vi "Traj_constraint_encapsulate.vi"() -> ()   [LabVIEW 2019]
uses:
  <vilib>/Utility/Data Type/Type Definitions/Data Type.ctl
  <vilib>/Utility/Data Type/Type Definitions/Type Definition Info.ctl
  <vilib>/Rock Robotics/WPI/ThirdParty/JAS_Junk/TrajLib/POSE2D.ctl
  <vilib>/Rock Robotics/WPI/ThirdParty/JAS_Junk/TrajLib/TRANSLATION2D.ctl
  <vilib>/Rock Robotics/WPI/ThirdParty/JAS_Junk/TrajLib/ROTATION2D.ctl
  <vilib>/Rock Robotics/WPI/ThirdParty/JAS_Junk/TrajLib/SIMPLE_MOTOR_FF.ctl
  <vilib>/Rock Robotics/WPI/ThirdParty/JAS_Junk/TrajLib/TRAJ_CONSTRAINT_DIIF_DRIVE_KINEMATICS.ctl
  <vilib>/Rock Robotics/WPI/ThirdParty/JAS_Junk/TrajLib/DIFF_DRIVE_KINEMATICS.ctl
  <vilib>/Rock Robotics/WPI/ThirdParty/JAS_Junk/TrajLib/TRAJ_CONSTRAINT_CENTRIPETAL_ACCEL.ctl
  <vilib>/Rock Robotics/WPI/ThirdParty/JAS_Junk/TrajLib/TRAJ_CONSTRAINT_DIIF_DRIVE_VOLTAGE.ctl
  <vilib>/Rock Robotics/WPI/ThirdParty/JAS_Junk/TrajLib/TRAJ_CONSTRAINT_MECA_DRIVE_KINEMATICS.ctl
  <vilib>/Rock Robotics/WPI/ThirdParty/JAS_Junk/TrajLib/MECA_DRIVE_KINEMATICS.ctl
  <vilib>/Analysis/Matrix/Datatypes/RealMatrix.ctl
  <vilib>/Rock Robotics/WPI/ThirdParty/JAS_Junk/TrajLib/TRAJ_CONSTRAINT_SWERVE_DRIVE_KINEMATICS.ctl
  <vilib>/Rock Robotics/WPI/ThirdParty/JAS_Junk/TrajLib/SWERVE_DRIVE_KINEMATICS.ctl
  <vilib>/Rock Robotics/SystemInterfaces/NetworkCommunication/NetComm_UsageReport_report.vi
  <vilib>/Rock Robotics/WPI/ThirdParty/JAS_Junk/TrajLib/Util_LibraryGlobals.vi
  <vilib>/Rock Robotics/WPI/ThirdParty/JAS_Junk/TrajLib/Trajectory_Library.lvlib
  <vilib>/Analysis/Matrix/NI_Matrix.lvlib
  <vilib>/Utility/Data Type/NI_Data Type.lvlib
panel:
  out "error out":errorcluster
  out "Max Vel":dbl[](array[numeric])
  in  "Velocity":dbl
  in  "Curvature":dbl
  in  "statePose":T1={"TRANSLATION"={"X"=0.0, "Y"=0.0}, "ROTATION"={"VALUE"=0.0, "COS"=1.0, "SIN"=0.0}} {"ROTATION"."SIN" format="%13.4f"; "ROTATION"."COS" format="%13.4f"; "ROTATION"."VALUE" format="%13.4f"; "TRANSLATION"."Y" format="%14.3f"; "TRANSLATION"."X" format="%14.3f"}
  out "TypeDefInfo":T4[](array[typedef])
  out "TypeDef":bool[](array[boolean])
  out "Name":string[](array[string])
  out "Type":T5[](array[typedef])
  out "output array":variant[](array[variant])
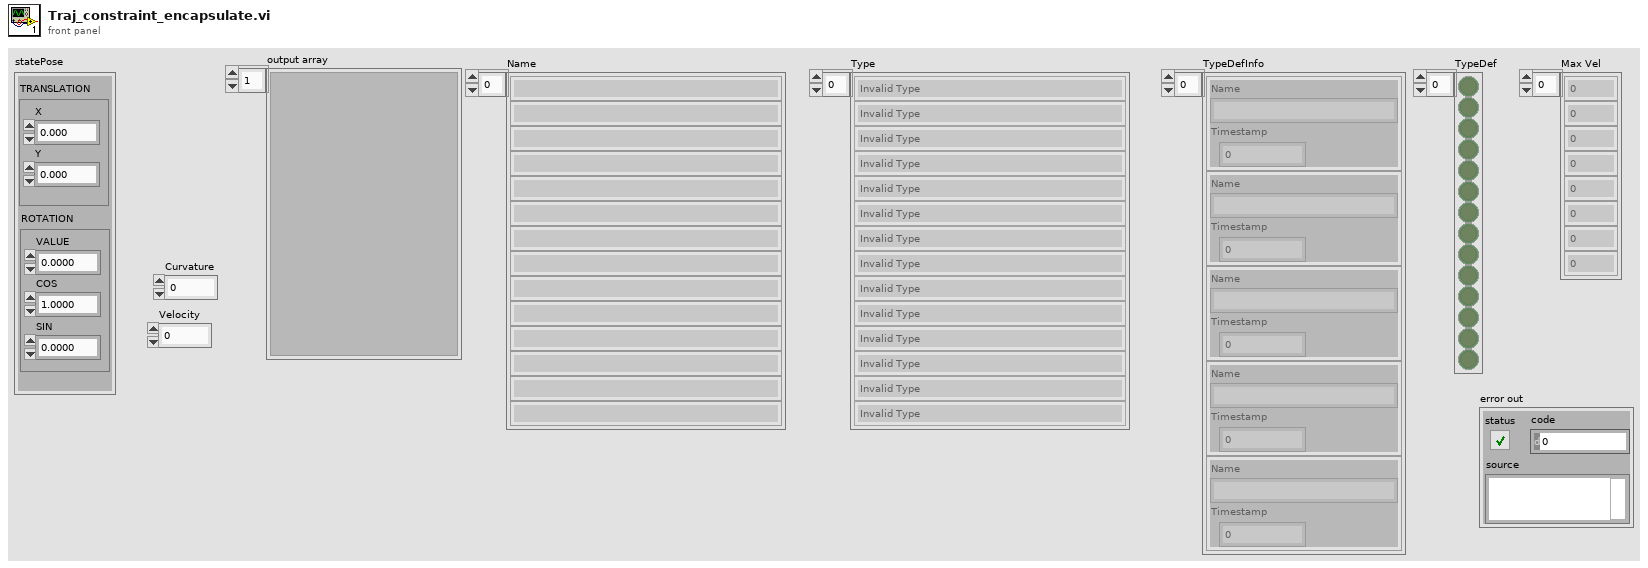
[diagram p1: front panel]
types:
  T1 = typedef "Trajectory_Library.lvlib/POSE2D.ctl" = cluster{"TRANSLATION":T2, "ROTATION":T3}
  T2 = typedef "Trajectory_Library.lvlib/TRANSLATION2D.ctl" = cluster{"X":dbl, "Y":dbl}
  T3 = typedef "Trajectory_Library.lvlib/ROTATION2D.ctl" = cluster{"VALUE":dbl, "COS":dbl, "SIN":dbl}
  T4 = typedef "NI_Data Type.lvlib/Type Definition Info.ctl" = cluster{"Name":string, "Timestamp":u32}
  T5 = typedef "NI_Data Type.lvlib/Data Type.ctl" = enum8{"Invalid Type", "Void", "I8", "I16", "I32", "I64", "U8", "U16", "U32", "U64", "Single Float", "Double Float", "Extended Float", "Single Complex", "Double Complex", "Extended Complex", "Enum U8", "Enum U16", "Enum U32", "Enum U64", "Single Float With Unit", "Double Float With Unit", "Extended Float With Unit", "Single Complex with Unit", "Double Complex with Unit", "Extended Complex with Unit", "Boolean", "String", "Path", "Picture", "Tag", "Array", "Cluster", "Variant", "LV Variant", "Waveform", "Timestamp", "Digital Waveform", "Digital Data", "ExpressData", "Refnum", "External Data", "VI", "Poly VI", "LabVIEW Class Instance", "Fixed Point", "Set Collection", "Map Collection"}
  T6 = typedef "Trajectory_Library.lvlib/SIMPLE_MOTOR_FF.ctl" = cluster{"Ks":dbl, "Kv":dbl, "Ka":dbl}
  T7 = typedef "Trajectory_Library.lvlib/MECA_DRIVE_KINEMATICS.ctl" = cluster{"FrontLeft":T2, "FrontRight":T2, "RearLeft":T2, "RearRight":T2, "InverseKinematics":T8, "ForwardKinematics":T8, "PrevCoR":T2}
  T8 = typedef "NI_Matrix.lvlib/RealMatrix.ctl" = dbl[][]
  T9 = typedef "Trajectory_Library.lvlib/SWERVE_DRIVE_KINEMATICS.ctl" = cluster{"NumModules":i32, "InverseKinematics":T8, "ForwardKinematics":T8, "Modules":T2[], "PrevCoR":T2}
  T10 = typedef "Trajectory_Library.lvlib/DIFF_DRIVE_KINEMATICS.ctl" = cluster{"TrackWidth_Meters":dbl}
  T11 = typedef "Trajectory_Library.lvlib/TRAJ_CONSTRAINT_MECA_DRIVE_KINEMATICS.ctl" = cluster{"Max Speed (M/S)":dbl, "MECA_DRIVE_KINEMATICS":T7}
  T12 = typedef "Trajectory_Library.lvlib/TRAJ_CONSTRAINT_SWERVE_DRIVE_KINEMATICS.ctl" = cluster{"Max Speed (M/S)":dbl, "SwerveKinematics":T9}
  T13 = typedef "Trajectory_Library.lvlib/TRAJ_CONSTRAINT_DIIF_DRIVE_VOLTAGE.ctl" = cluster{"Max Voltage":dbl, "DIFF_DRIVE_KINEMATICS":T10, "SIMPLE_MOTOR_FF":T6}
  T14 = typedef "Trajectory_Library.lvlib/TRAJ_CONSTRAINT_CENTRIPETAL_ACCEL.ctl" = cluster{"Max Cent Accel":dbl}
  T15 = typedef "Trajectory_Library.lvlib/TRAJ_CONSTRAINT_DIIF_DRIVE_KINEMATICS.ctl" = cluster{"Max Speed (M/S)":dbl, "DIFF_DRIVE_KINEMATICS":T10, "Max Accel (M/S2)":dbl}
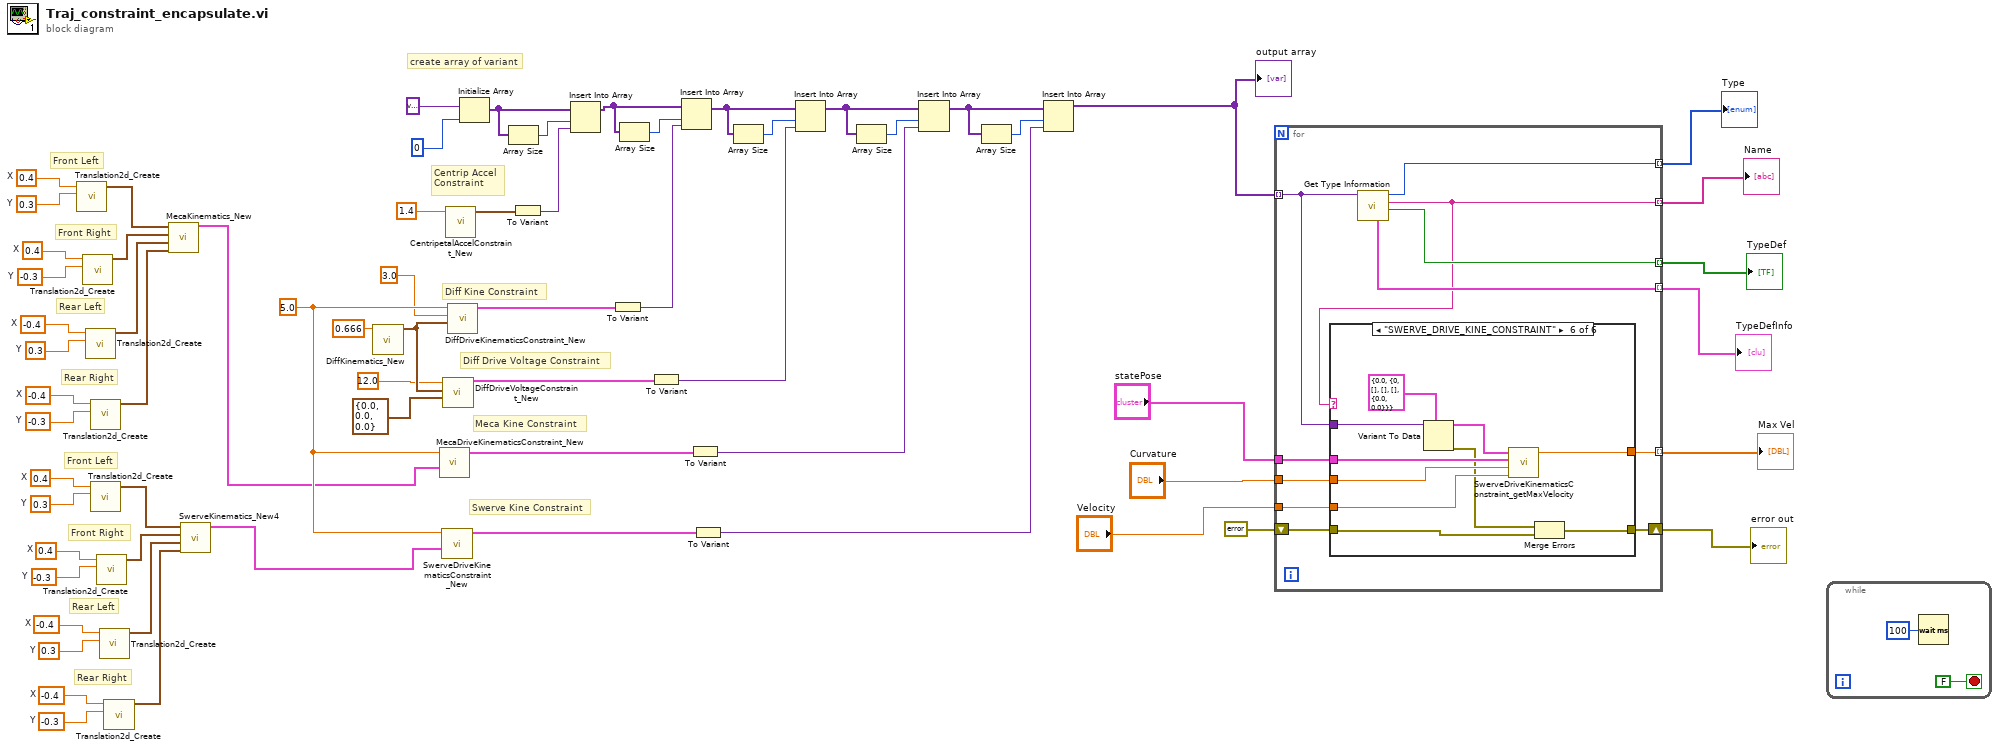
[diagram p0: block diagram]
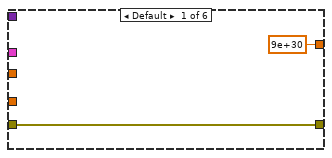
[diagram p2: hidden frame]
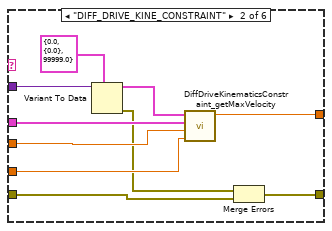
[diagram p3: hidden frame]
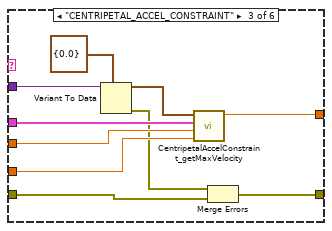
[diagram p4: hidden frame]
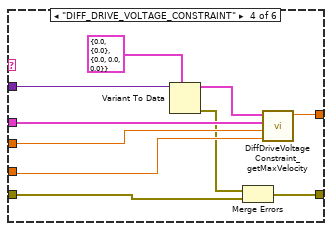
[diagram p5: hidden frame]
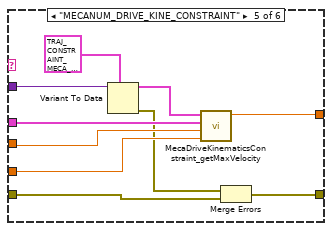
[diagram p6: hidden frame]
diagram:
  w10 = -0.4  # X
  w9 = -0.3  # Y
  w8 = -0.4  # X
  w7 = 0.3  # Y
  w6 = 0.4  # X
  w5 = -0.3  # Y
  w4 = 0.4  # X
  w3 = 0.3  # Y
  w23 = -0.4  # X
  w22 = -0.3  # Y
  w21 = -0.4  # X
  w20 = 0.3  # Y
  w19 = 0.4  # X
  w18 = -0.3  # Y
  w17 = 0.4  # X
  w16 = 0.3  # Y
  w51 = 5.0 ("Max Speed (M/S)")
  # "Rear Right"
  # "Rear Left"
  # "Front Right"
  # "Front Left"
  # "Rear Right"
  # "Rear Left"
  # "Front Right"
  # "Front Left"
  # "Swerve Kine Constraint"
  # "Meca Kine Constraint"
  # "Diff Drive Voltage Constraint"
  # "Diff Kine Constraint"
  # "Centrip Accel\nConstraint"
  # "create array of variant"
  n1 = call <vilib>:"Translation2d_Create.vi"("Y"=w3, "X"=w4) -> ("TRANSLATION"=w11:T2)  [unwired: 9 in]
  n2 = call <vilib>:"Translation2d_Create.vi"("Y"=w5, "X"=w6) -> ("TRANSLATION"=w12:T2)  [unwired: 9 in]
  n3 = call <vilib>:"Translation2d_Create.vi"("Y"=w7, "X"=w8) -> ("TRANSLATION"=w13:T2)  [unwired: 9 in]
  n4 = call <vilib>:"Translation2d_Create.vi"("Y"=w9, "X"=w10) -> ("TRANSLATION"=w14:T2)  [unwired: 9 in]
  n5 = call <vilib>:"Translation2d_Create.vi"("Y"=w16, "X"=w17) -> ("TRANSLATION"=w24:T2)  [unwired: 9 in]
  n6 = call <vilib>:"Translation2d_Create.vi"("Y"=w18, "X"=w19) -> ("TRANSLATION"=w25:T2)  [unwired: 9 in]
  n7 = call <vilib>:"Translation2d_Create.vi"("Y"=w20, "X"=w21) -> ("TRANSLATION"=w26:T2)  [unwired: 9 in]
  n8 = call <vilib>:"Translation2d_Create.vi"("Y"=w22, "X"=w23) -> ("TRANSLATION"=w27:T2)  [unwired: 9 in]
  n9 = call <vilib>:"MecaKinematics_New.vi"("RearRight"=w14, "RearLeft"=w13, "FrontRight"=w12, "FrontLeft"=w11) -> ("MECA_DRIVE_KINEMATICS"=w2:T7)  [unwired: 7 in]
  n10 = call <vilib>:"SwerveKinematics_New4.vi"("wheel 3"=w27, "wheel 2"=w26, "wheel 1"=w25, "wheel 0"=w24) -> ("SWERVE_DRIVE_KINEMATICS"=w15:T9)  [unwired: 7 in]
  n11 = call <vilib>:"DiffKinematics_New.vi"("TrackWidth_Meters"=0.666) -> ("DIFF_DRIVE_KINEMATICS"=w52:T10)  [unwired: 10 in]
  n12 = call <vilib>:"MecaDriveKinematicsConstraint_New.vi"("MecanumKinematics"=w2, "Max Speed (M/S)"=w51) -> ("MECANUM_DRIVE_KINE_CONSTRAINT"=w41:T11)  [unwired: 9 in]
  n13 = call <vilib>:"SwerveDriveKinematicsConstraint_New.vi"("SwerveKinematics"=w15, "Max Speed (M/S)"=w51) -> ("SWERVE_DRIVE_KINE_CONSTRAINT"=w40:T12)  [unwired: 9 in]
  n14 = call <vilib>:"DiffDriveVoltageConstraint_New.vi"("SIMPLE_MOTOR_FF"=T6 {"Ks"=0.0, "Kv"=0.0, "Ka"=0.0}, "DIFF_DRIVE_KINEMATICS"=w52, "Max Voltage"=12.0) -> ("DIFF_DRIVE_VOLTAGE_CONSTRAINT"=w39:T13)  [unwired: 8 in]
  n15 = call <vilib>:"CentripetalAccelConstraint_New.vi"("Max Cent Accel"=1.4) -> ("CENTRIPETAL_ACCEL_CONSTRAINT"=w43:T14)  [unwired: 10 in]
  n16 = call <vilib>:"DiffDriveKinematicsConstraint_New.vi"("DIFF_DRIVE_KINEMATICS"=w52, "Max Accel (M/S2)"=3.0, "Max Speed (M/S)"=w51) -> ("DIFF_DRIVE_KINE_CONSTRAINT"=w38:T15)  [unwired: 8 in]
  n17 = Initialize Array(variant, 0 ("dimension size")) -> (w64:variant[])
  n18 = Array Size(array=w64) -> (size(s)=w63:i32)
  n19 = To Variant(anything=w43) -> (Variant=w42:variant)
  n20 = Insert Into Array(array=w64, index=w63, new element=w42) -> (w58:variant[])
  n21 = To Variant(anything=w38) -> (Variant=w37:variant)
  n22 = Array Size(array=w58) -> (size(s)=w62:i32)
  n23 = To Variant(anything=w39) -> (Variant=w36:variant)
  n24 = Insert Into Array(array=w58, index=w62, new element=w37) -> (w57:variant[])
  n25 = To Variant(anything=w41) -> (Variant=w35:variant)
  n26 = To Variant(anything=w40) -> (Variant=w34:variant)
  n27 = Array Size(array=w57) -> (size(s)=w61:i32)
  n28 = Insert Into Array(array=w57, index=w61, new element=w36) -> (w56:variant[])
  n29 = Array Size(array=w56) -> (size(s)=w60:i32)
  n30 = Insert Into Array(array=w56, index=w60, new element=w35) -> (w55:variant[])
  n31 = Array Size(array=w55) -> (size(s)=w59:i32)
  n32 = Insert Into Array(array=w55, index=w59, new element=w34) -> (w48:variant[])
  "output array" <- w48
  n33 = for {
    tunnel: w48 -> [w73] mode=indexing
    tunnel: [w77] -> w47 mode=indexing
    tunnel: [w74] -> w46 mode=indexing
    tunnel: [w75] -> w45 mode=indexing
    tunnel: [w76] -> w44 mode=indexing
    tunnel: "statePose" -> [w72]
    tunnel: "Curvature" -> [w71]
    tunnel: "Velocity" -> [w70]
    tunnel: [w69] -> w30 mode=indexing
    shift-right: [w68] -> w29
    shift-left: errorcluster {"status"=FALSE, "code"=0, "source"=""} ("error out") -> [w67]
    n34 = call <vilib>:"Get Type Information.vi"("variant"=w73) -> ("type definition"=w75:bool, "name"=w74:string, "type"=w77:T5, "type definition info"=w76:T4)  [unwired: 6 in, 1 out]
    n35 = case shown="\"SWERVE_DRIVE_KINE_CONSTRAINT\"" w74 {
      tunnel: w73 -> [_ w88 w97 w103 w116 w127]
      tunnel: w72 -> [_ w86 w95 w106 w115 w125]
      tunnel: w71 -> [_ w85 w94 w105 w114 w124]
      tunnel: w70 -> [_ w84 w93 w104 w113 w123]
      tunnel: [9e+30 ("absMaxVelocity") w83 w96 w107 w117 w126] -> w69
      tunnel: [w78 w81 w92 w101 w112 w122] -> w68
      tunnel: w67 -> [w78 w80 w90 w100 w110 w120]
      frame Default {
      }
      frame "DIFF_DRIVE_KINE_CONSTRAINT" {
        n36 = Variant To Data(type=T15 {"Max Speed (M/S)"=0.0, "DIFF_DRIVE_KINEMATICS"={"TrackWidth_Meters"=0.0}, "Max Accel (M/S2)"=99999.0} ("DIFF_DRIVE_KINE_CONSTRAINT"), Variant=w88) -> (data=w87:T15, error out=w82:errorcluster)  [unwired: 1 in]
        n37 = call <vilib>:"DiffDriveKinematicsConstraint_getMaxVelocity.vi"("Velocity"=w84, "Curvature"=w85, "statePose"=w86, "DIFF_DRIVE_KINE_CONSTRAINT"=w87) -> ("absMaxVelocity"=w83:dbl)  [unwired: 7 in]
        n38 = Merge Errors(w82, w80) -> (w81:errorcluster)
      }
      frame "CENTRIPETAL_ACCEL_CONSTRAINT" {
        n39 = Variant To Data(type=T14 {"Max Cent Accel"=0.0} ("CENTRIPETAL_ACCEL_CONSTRAINT"), Variant=w97) -> (data=w98:T14, error out=w91:errorcluster)  [unwired: 1 in]
        n40 = call <vilib>:"CentripetalAccelConstraint_getMaxVelocity.vi"("Velocity"=w93, "Curvature"=w94, "statePose"=w95, "CENTRIPETAL_ACCEL_CONSTRAINT"=w98) -> ("absMaxVelocity"=w96:dbl)  [unwired: 7 in]
        n41 = Merge Errors(w91, w90) -> (w92:errorcluster)
      }
      frame "DIFF_DRIVE_VOLTAGE_CONSTRAINT" {
        n42 = Variant To Data(type=T13 {"Max Voltage"=0.0, "DIFF_DRIVE_KINEMATICS"={"TrackWidth_Meters"=0.0}, "SIMPLE_MOTOR_FF"={"Ks"=0.0, "Kv"=0.0, "Ka"=0.0}} ("DIFF_DRIVE_VOLTAGE_CONSTRAINT"), Variant=w103) -> (data=w108:T13, error out=w102:errorcluster)  [unwired: 1 in]
        n43 = Merge Errors(w102, w100) -> (w101:errorcluster)
        n44 = call <vilib>:"DiffDriveVoltageConstraint_getMaxVelocity.vi"("Velocity"=w104, "Curvature"=w105, "statePose"=w106, "DIFF_DRIVE_VOLTAGE_CONSTRAINT"=w108) -> ("absMaxVelocity"=w107:dbl)  [unwired: 7 in]
      }
      frame "MECANUM_DRIVE_KINE_CONSTRAINT" {
        n45 = Variant To Data(type=T11 {"Max Speed (M/S)"=0.0, "MECA_DRIVE_KINEMATICS"={"FrontLeft"={"X"=0.0, "Y"=0.0}, "FrontRight"={"X"=0.0, "Y"=0.0}, "RearLeft"={"X"=0.0, "Y"=0.0}, "RearRight"={"X"=0.0, "Y"=0.0}, "InverseKinematics"=[[0.0, 1.0, -1.0, 0.0], [0.0, 1.0, 1.0, 0.0], [0.0, 1.0, 1.0, 0.0], [0.0, 1.0, -1.0, 0.0]], "ForwardKinematics"=[[0.0, 1.0, -1.0, 0.0], [0.0, 1.0, 1.0, 0.0], [0.0, 1.0, 1.0, 0.0], [0.0, 1.0, -1.0, 0.0]], "PrevCoR"={"X"=0.0, "Y"=0.0}}} ("MECANUM_DRIVE_KINE_CONSTRAINT"), Variant=w116) -> (data=w118:T11, error out=w111:errorcluster)  [unwired: 1 in]
        n46 = call <vilib>:"MecaDriveKinematicsConstraint_getMaxVelocity.vi"("Velocity"=w113, "Curvature"=w114, "statePose"=w115, "MECANUM_DRIVE_KINE_CONSTRAINT"=w118) -> ("absMaxVelocity"=w117:dbl)  [unwired: 7 in]
        n47 = Merge Errors(w111, w110) -> (w112:errorcluster)
      }
      frame "SWERVE_DRIVE_KINE_CONSTRAINT" {
        n48 = Variant To Data(type=T12 {"Max Speed (M/S)"=0.0, "SwerveKinematics"={"NumModules"=0, "InverseKinematics"=[], "ForwardKinematics"=[], "Modules"=[], "PrevCoR"={"X"=0.0, "Y"=0.0}}} ("SWERVE_DRIVE_KINE_CONSTRAINT"), Variant=w127) -> (data=w128:T12, error out=w121:errorcluster)  [unwired: 1 in]
        n49 = call <vilib>:"SwerveDriveKinematicsConstraint_getMaxVelocity.vi"("Velocity"=w123, "Curvature"=w124, "statePose"=w125, "SWERVE_DRIVE_KINE_CONSTRAINT"=w128) -> ("absMaxVelocity"=w126:dbl)  [unwired: 7 in]
        n50 = Merge Errors(w121, w120) -> (w122:errorcluster)
      }
    }
  }
  "Type" <- w47
  "Name" <- w46
  "TypeDef" <- w45
  "TypeDefInfo" <- w44
  "Max Vel" <- w30
  "error out" <- w29
  n51 = while {
    stop <- FALSE stop-if-true
    n52 = Wait (ms)(milliseconds to wait=u32 100) -> ()  [unwired: 1 out]
  }
